vi "Close.vi"(8 "error in (no error)":errorcluster, 11 "NI Scope in":refnum<class "NI Scope.lvclass">) -> (0 "error out":errorcluster, 3 "NI Scope out":refnum<class "NI Scope.lvclass">)   [LabVIEW 2025, in "Scope.lvlib" / "NI Scope.lvclass"]
uses:
  NI Scope.lvclass
  NI Scope.lvclass/NI Scope.ctl
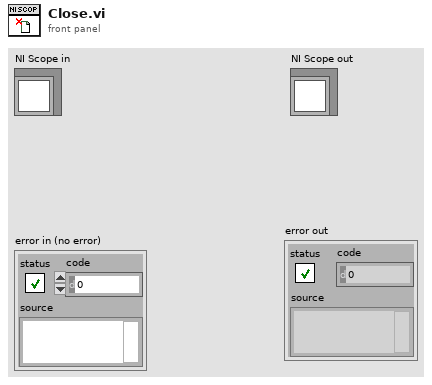
[diagram p1: front panel]
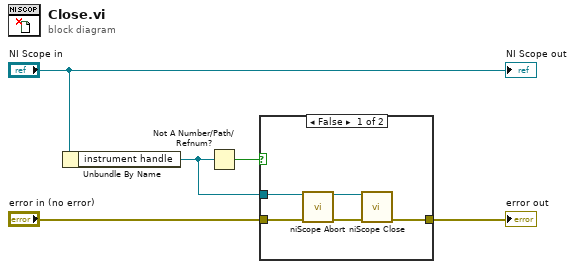
[diagram p0: block diagram]
diagram:
  n1 = Unbundle By Name("NI Scope in") -> ("instrument handle"=w2:refnum<k15>)
  n2 = Not A Number/Path/Refnum?(number/path/refnum=w2) -> (NaN/Path/Refnum?=w1:bool)
  n3 = case shown="False" w1 {
    tunnel: [w10 w11] -> w5
    tunnel: "error in (no error)" -> [w9 w11]
    tunnel: w2 -> [w6 _]
    frame False {
      n4 = call <instrlib>:"niScope Abort.vi"("instrument handle"=w6, "error in"=w9) -> ("instrument handle out"=w7:refnum<k15>, "error out"=w8:errorcluster)  [unwired: 12 in]
      n5 = call <instrlib>:"niScope Close.vi"("instrument handle"=w7, "error in"=w8) -> ("error out"=w10:errorcluster)  [unwired: 13 in]
    }
    frame True {
    }
  }
  "error out" <- w5
  "NI Scope out" <- "NI Scope in"
